vi "_Read Spreadsheet.vi"(0 "Start Path":path=path "C:/") -> (1 "Column Titles":string[](array[string]), 2 "Imported Table":string[][](array[string]), 3 "Table":T1[](array[typedef]), 4 "Succeded":bool)   [LabVIEW 2012]
uses:
  Type/_RT Configuration 2.ctl
  <vilib>/Utility/file.llb/Read From Spreadsheet File (string).vi
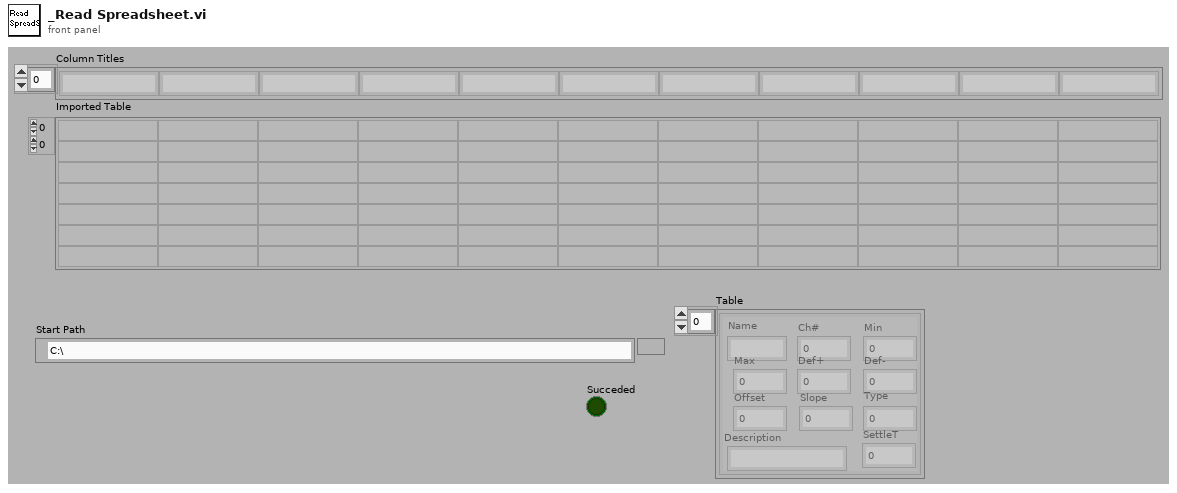
[diagram p1: front panel]
types:
  T1 = typedef "_RT Configuration 2.ctl" = cluster{"Name":string, "Ch#":u8, "Min":dbl, "Max":dbl, "Def+":dbl, "Def-":dbl, "Offset":dbl, "Slope":dbl, "Type":u8, "Description":string, "SettleT":dbl}
  T2 = enum32{"existing file", "new file", "new or existing file", "existing dir", "new dir", "new or existing dir", "existing file (use LLBs)", "new file (use LLBs)", "new or existing file (use LLBs)", "new or existing file or directory (use LLBs)"}
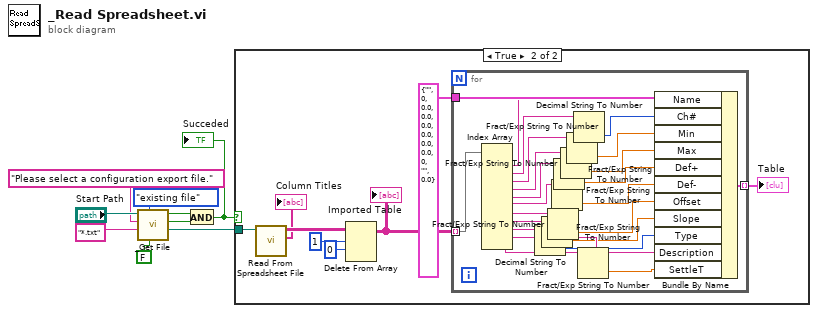
[diagram p0: block diagram]
diagram:
  n1 = call "_Get File.vi"("For Write (T)"=FALSE, "select mode (new or existing)"=T2."existing file", "extension (isd)"="*.txt" ("pattern (all files)"), "prompt"="Please select a configuration export file.", "Start Path"="Start Path") -> ("Seleted File"=w4:path, "Exists"=w2:bool, "Succeeded"=w3:bool)  [unwired: 1 in, 1 out]
  n2 = And(x=w3, y=w2) -> (x .and. y?=w1:bool)
  "Succeded" <- w1
  n3 = case shown="True" w1 {
    tunnel: w4 -> [_ w15]
    frame False {
    }
    frame True {
      n4 = call-poly <vilib>:"Read From Spreadsheet File.vi"("file path (dialog if empty)"=w15) -> ("first row"=→"Column Titles":string[], "all rows"=w11:string[][])  [unwired: 6 in, 3 out]
      n5 = Delete From Array(array=w11, length=1, index (row)=0) -> (array with subset deleted=w14:string[][])  [unwired: 1 in, 1 out]
      "Imported Table" <- w14
      n6 = for {
        tunnel: w14 -> [w40] mode=indexing
        tunnel: T1 {"Name"="", "Ch#"=0, "Min"=0.0, "Max"=0.0, "Def+"=0.0, "Def-"=0.0, "Offset"=0.0, "Slope"=0.0, "Type"=0, "Description"="", "SettleT"=0.0} ("Configuration") -> [w35]
        tunnel: [w27] -> w12 mode=indexing
        n7 = Index Array(array=w40) -> (element #1=w34:string, element #2=w39:string, element #3=w38:string, element #4=w37:string, element #5=w36:string, element #6=w23:string, element #7=w25:string, element #8=w24:string, element #9=w22:string, element #10=w21:string, element #11=w19:string)  [unwired: 11 in]
        n8 = Decimal String To Number(string=w22) -> (number=w28:i32)  [unwired: 3 out]
        n9 = Fract/Exp String To Number(string=w24) -> (number=w20:dbl)  [unwired: 4 out]
        n10 = Fract/Exp String To Number(string=w25) -> (number=w29:dbl)  [unwired: 4 out]
        n11 = Fract/Exp String To Number(string=w23) -> (number=w26:dbl)  [unwired: 4 out]
        n12 = Fract/Exp String To Number(string=w36) -> (number=w30:dbl)  [unwired: 4 out]
        n13 = Fract/Exp String To Number(string=w37) -> (number=w31:dbl)  [unwired: 4 out]
        n14 = Fract/Exp String To Number(string=w38) -> (number=w32:dbl)  [unwired: 4 out]
        n15 = Decimal String To Number(string=w39) -> (number=w33:i32)  [unwired: 3 out]
        n16 = Fract/Exp String To Number(string=w19) -> (number=w18:dbl)  [unwired: 4 out]
        n17 = Bundle By Name(cluster=w35, "Name"=w34, "Ch#"=w33, "Min"=w32, "Max"=w31, "Def+"=w30, "Def-"=w26, "Offset"=w29, "Slope"=w20, "Type"=w28, "Description"=w21, "SettleT"=w18) -> (w27:T1)
      }
      "Table" <- w12
    }
  }
